vi "Link Dependencies.vi"   [LabVIEW 2017, in "libssh2.lvlib"]
uses:
  libssh2.lvlib
  libssl-4-x64.dll
  libcrypto-4-x64.dll
  libssl-4.dll
  libcrypto-4.dll
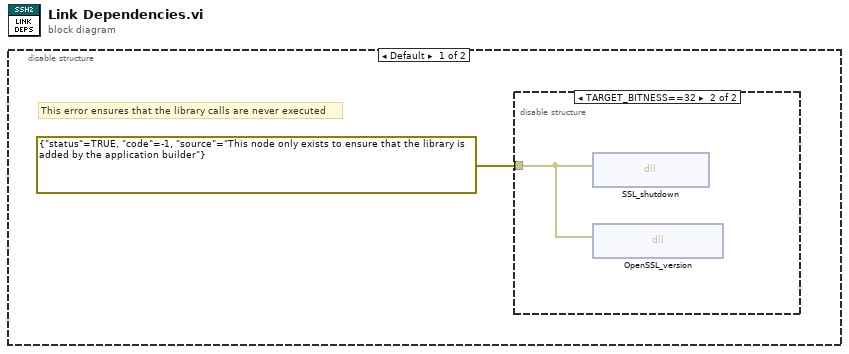
[diagram p0: block diagram]
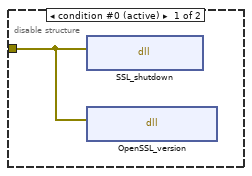
[diagram p2: hidden frame]
diagram:
  n1 = disable-structure shown="Default" {
    frame condition #0 (active) {
      # "This error ensures that the library calls are never executed"
      n2 = disable-structure shown="TARGET_BITNESS==32" {
        disable-tunnel: errorcluster {"status"=TRUE, "code"=-1, "source"="This node only exists to ensure that the library is added by the application builder"} ("error in (no error)") -> [w2 w3]
        frame condition #0 (active) {
          n3 = dll-call lib="C:/Users/Pascal/Projects/Home/lvssh2/libssh2/libssl-4-x64.*" fn="SSL_shutdown"(error in=w2) -> ()  [unwired: 3 in, 2 out]
          n4 = dll-call lib="C:/Users/Pascal/Projects/Home/lvssh2/libssh2/libcrypto-4-x64.*" fn="OpenSSL_version"(error in=w2) -> ()  [unwired: 3 in, 2 out]
        }
        frame condition #1 {
          n5 = dll-call lib="C:/Users/Pascal/Projects/Home/lvssh2/libssh2/libssl-4.*" fn="SSL_shutdown"(error in=w3) -> ()  [unwired: 3 in, 2 out]
          n6 = dll-call lib="C:/Users/Pascal/Projects/Home/lvssh2/libssh2/libcrypto-4.*" fn="OpenSSL_version"(error in=w3) -> ()  [unwired: 3 in, 2 out]
        }
      }
    }
    frame condition #1 {
    }
  }
